vi "FTW-TestExecutive-Core_Initialize.vi"(0 "Test Executive":refnum<class "FTW-TestExecutive-Core.lvclass">, 5 "Initialization Sequence":string, 7 "FTW Actor Instance Configuration":string, 11 "error in (no error)":errorcluster) -> (4 "FTW-TestExecutive-Core Out":refnum<class "FTW-TestExecutive-Core.lvclass">, 6 "Event Refnums":T1, 10 "Refresh Period":dbl, 15 "error out":errorcluster)   [LabVIEW 2018, in "FTW-TestExecutive-Core.lvclass"]
uses:
  FTW-TestExecutive-Core.lvclass
  Message/Request/FTW-Message-IncomingRequest.lvclass
  Message/Base/FTW-Message.lvclass
  FTW-TestExecutive-Core.lvclass/FTW-TestExecutive-Core.ctl
  6bec97a4-0dc4-4e28-af4a-dd3c190fc740.vi
  JSON/core/FTW-JSON-Core-EncodingFlags.vi
  Reflection/FTW-Reflection-Type.vi
  JSON/FTW-JSON-Parse.vi
  container/FTW-Container-GetFlattenedValue.vi
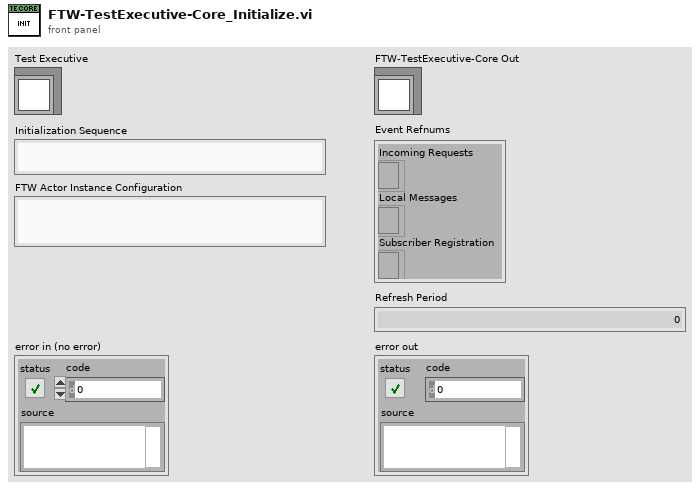
[diagram p1: front panel]
types:
  T1 = cluster{"Incoming Requests":refnum<event-registration>, "Local Messages":refnum<event-registration>, "Subscriber Registration":refnum<event-registration>}
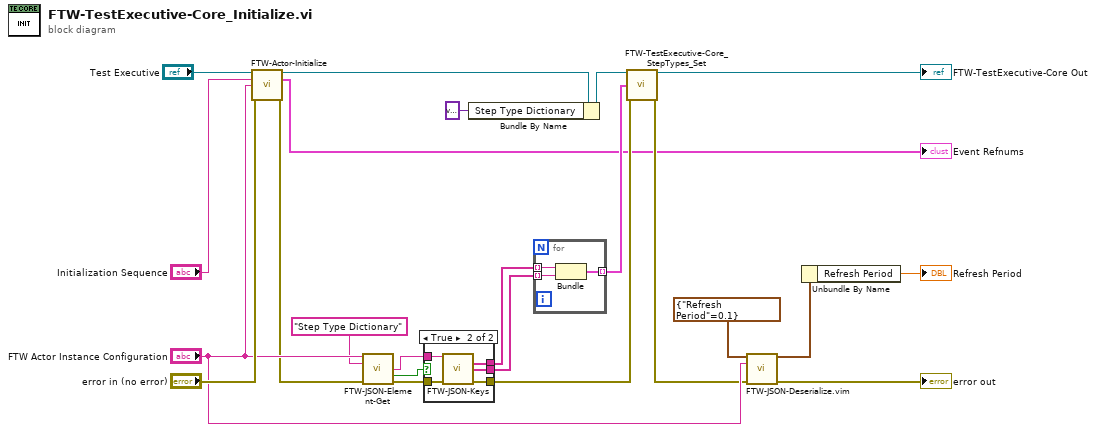
[diagram p0: block diagram]
diagram:
  n1 = call-dynamic "FTW-Actor-Initialize.vi"("FTW Actor Instance Type"="Test Executive", "Initialization Job Sequence"="Initialization Sequence", "Actor Instance Configuration"="FTW Actor Instance Configuration", "error in"="error in (no error)") -> ("FTW Actor Instance"=w8:refnum<class "FTW-TestExecutive-Core.lvclass">, "Event Refnums"=→"Event Refnums":T1, "error out"=w12:errorcluster)  [unwired: 9 in]
  n2 = call "FTW-JSON-Element-Get.vi"("JSON Opject"="FTW Actor Instance Configuration", "Key"="Step Type Dictionary", "error in"=w12) -> ("Element"=w14:string, "Found?"=w2:bool, "error out"=w13:errorcluster)  [unwired: 10 in]
  n3 = case shown="True" w2 {
    tunnel: w14 -> [_ w29]
    tunnel: w13 -> [w24 w28]
    tunnel: [_ w27] -> w11
    tunnel: [_ w26] -> w10
    tunnel: [w24 w25] -> w4
    frame False {
    }
    frame True {
      n4 = call "FTW-JSON-Keys.vi"("JSON Opject"=w29, "error in"=w28) -> ("Keys"=w27:string[], "Values"=w26:string[], "error out"=w25:errorcluster)  [unwired: 11 in]
    }
  }
  n5 = Bundle By Name(cluster=w8, "Step Type Dictionary"=variant) -> (w6:refnum<class "FTW-TestExecutive-Core.lvclass">)
  n6 = for {
    tunnel: w11 -> [w32] mode=indexing
    tunnel: w10 -> [w31] mode=indexing
    tunnel: [w30] -> w9 mode=indexing
    n7 = Bundle("String"=w32, "String"=w31) -> (w30:cluster{"String":string, "String":string})  [unwired: 1 in]
  }
  n8 = call "FTW-TestExecutive-Core_StepTypes_Set.vi"("FTW-TestExecutive-Core In"=w6, "Step Types"=w9, "error in"=w4) -> ("FTW-TestExecutive-Core Out"=→"FTW-TestExecutive-Core Out":refnum<class "FTW-TestExecutive-Core.lvclass">, "error out"=w3:errorcluster)  [unwired: 11 in]
  n9 = call "FTW-JSON-Deserialize.vim"("Type In"=cluster{"Refresh Period":dbl} {"Refresh Period"=0.1} ("Type and Defaults"), "JSON String"="FTW Actor Instance Configuration", "error in"=w3) -> ("Type Out"=w21:cluster{"Refresh Period":dbl}, "error out"=→"error out":errorcluster)  [unwired: 11 in]
  n10 = Unbundle By Name(w21) -> ("Refresh Period"=→"Refresh Period":dbl)
